vi "Execute.vi"(8 "error in (no error)":errorcluster, 9 "Parameters":map{string, variant}(c390), 10 "Query":string, 11 "Database Manager in":refnum<class "Database Manager.lvclass">) -> (0 "error out":errorcluster, 3 "Database Manager out":refnum<class "Database Manager.lvclass">)   [LabVIEW 2019, in "HierDAL Library.lvlib" / "Database.lvlib" / "Database Manager.lvclass"]
doc: "Executes a non-query SQL command (e.g., INSERT, UPDATE, DELETE).\nParameters are used to safely inject values into the SQL command, preventing SQL injection attacks.\nIt ensure that inputs are only ever treated as literal values and never executed.\n\nParameters can be prefixed with either :, @, or $.\ne.g.\n\"\"\"\n INSERT INTO user (name)\n VALUES ($name)\n\"\"\"\n\n<b>Query</b> - The SQL command to execute.\n<b>Parameters</b> - A map of parameter names (must contain the prefixes) and their corresponding values."
uses:
  Database Manager.lvclass
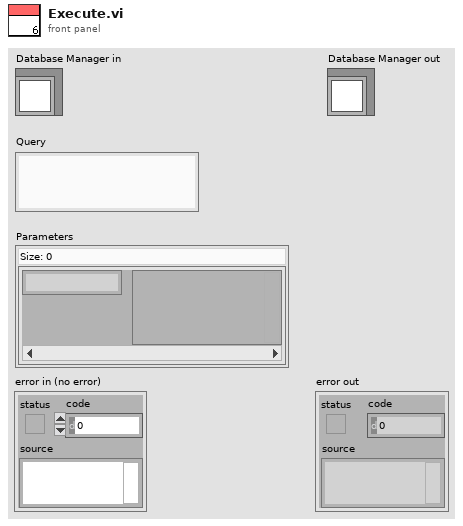
[diagram p1: front panel]
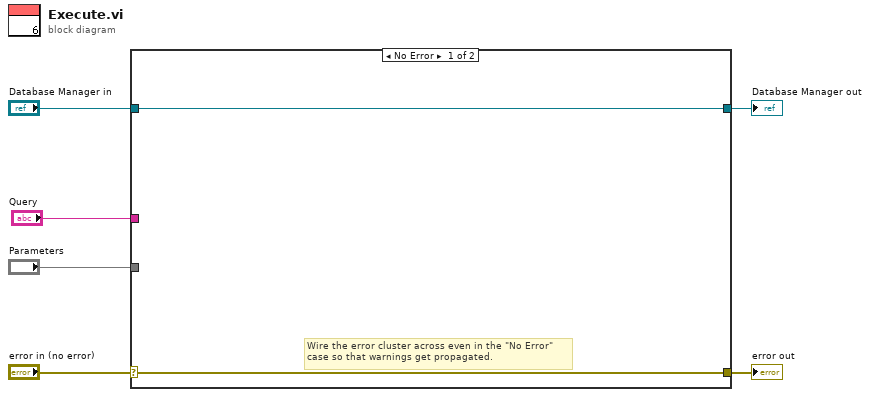
[diagram p0: block diagram]
diagram:
  n1 = case shown="No Error" "error in (no error)" {
    selector: "error in (no error)" -> [w7 w10]
    tunnel: [w7 w10] -> w5
    tunnel: [w8 w9] -> w3
    tunnel: "Database Manager in" -> [w8 w9]
    tunnel: "Query" -> [_ _]
    tunnel: "Parameters" -> [_ _]
    frame No Error {
      # "Wire the error cluster across even in the \"No Error\"\ncase so that warnings get propagated."
    }
    frame Error {
    }
  }
  "error out" <- w5
  "Database Manager out" <- w3
